vi "On Click Start Camera Calibration.vi"(8 "error in (no error)":errorcluster, 11 "App in":refnum<class "App.lvclass">) -> (0 "error out":errorcluster, 3 "App out":refnum<class "App.lvclass">)   [LabVIEW 2020, in "AR Example.lvlib" / "App.lvclass"]
uses:
  App.lvclass
  App.lvclass/App.ctl
  UI/UI.lvclass
  UI/Tab Control.ctl
  Timeout Action.ctl
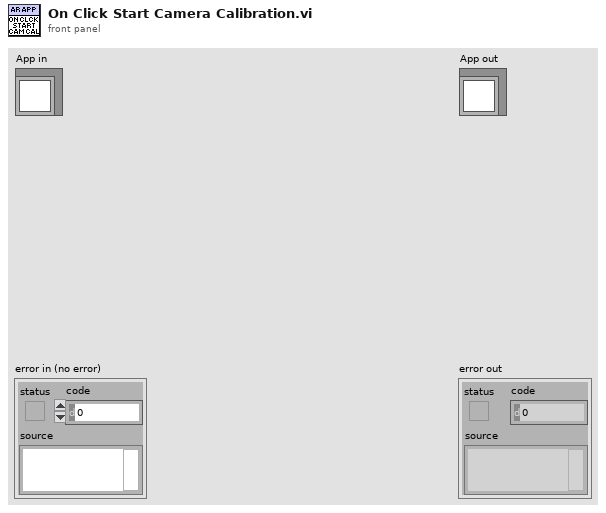
[diagram p1: front panel]
types:
  T1 = typedef "AR Example.lvlib/App.lvclass/Timeout Action.ctl" = enum16{"None", "Setup Camera Action", "Camera Calibration Action"}
  T2 = typedef "AR Example.lvlib/UI.lvclass/Tab Control.ctl" = enum8{"Config Load", "Camera Selection", "Camera Calibration"}
  T3 = typedef "g_ar_toolkit.common.lvlib/Image Size (Integer).ctl" = cluster{"Width":u16, "Height":u16}
  T4 = typedef "g_ar_toolkit.image.lvlib/Image Draw Offset.ctl" = cluster{"Left":i16, "Top":i16}
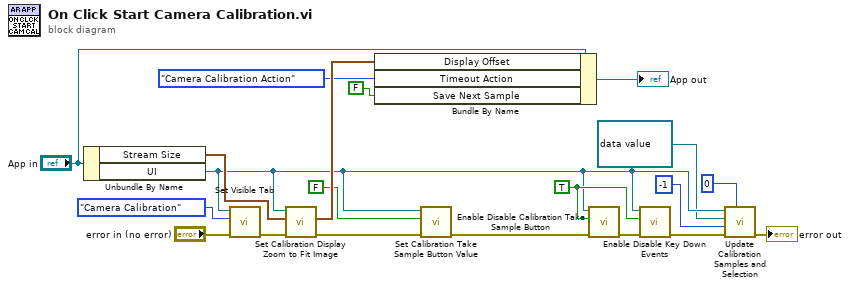
[diagram p0: block diagram]
diagram:
  w6 = TRUE ("Enable?")
  n1 = Unbundle By Name("App in") -> ("Stream Size"=w16:T3, "UI"=w4:refnum<class "UI.lvclass">)
  n2 = call-dynamic "Set Visible Tab.vi"("error in (no error)"="error in (no error)", "Value"=Tab_Control."Camera Calibration", "UI in"=w4) -> ("error out"=w19:errorcluster)  [unwired: 8 in]
  n3 = call-dynamic "Set Calibration Display Zoom to Fit Image.vi"("error in (no error)"=w19, "Size"=w16, "UI in"=w4) -> ("error out"=w17:errorcluster, "Offset"=w13:T4)  [unwired: 7 in]
  n4 = Bundle By Name(cluster="App in", "Display Offset"=w13, "Timeout Action"=Timeout_Action."Camera Calibration Action" ("Shared.Timeout Action"), "Save Next Sample"=FALSE ("Camera Calibration.Save Next Sample")) -> (→"App out":refnum<class "App.lvclass">)
  n5 = call-dynamic "Set Calibration Take Sample Button Value.vi"("error in (no error)"=w17, "Value"=FALSE, "UI in"=w4) -> ("error out"=w10:errorcluster)  [unwired: 8 in]
  n6 = call-dynamic "Enable Disable Calibration Take Sample Button.vi"("error in (no error)"=w10, "Enable?"=w6, "UI in"=w4) -> ("error out"=w8:errorcluster)  [unwired: 8 in]
  n7 = call "Enable Disable Key Down Events.vi"("error in (no error)"=w8, "Enable?"=w6, "UI in"=w4) -> ("error out"=w7:errorcluster)  [unwired: 8 in]
  n8 = call "Update Calibration Samples and Selection.vi"("N-Samples"=0, "error in (no error)"=w7, "Selection"=-1, "Sample"=refnum<data-value> refnum, "UI in"=w4) -> ("error out"=→"error out":errorcluster)  [unwired: 6 in]
